vi "Compare to Accel Distances.vi"(5 "dA":dbl, 6 "Sample Period (s)":dbl, 7 "Values":cluster{"accel":dbl, "velocity":dbl}, 8 "Speeds":T1={"maxV (fps)"=20.0, "Accel Limit (fps^2)"=20.0, "Initial V (fps)"=0.0, "Sample Period (s)"=0.02, "Jerk Limit (fps^3)"=0.0, "Front Distances"={"distance (ft)"=0.0, "baseline (ft)"=0.0, "high (ft)"=0.0}, "Back Distances"={"distance (ft)"=0.0, "baseline (ft)"=0.0, "high (ft)"=0.0}}, 10 "Current  Length":dbl, 11 "Total Segment Length":dbl) -> (0 "End Loop":bool, 1 "Ends":cluster{"Accel End":bool, "Decel End":bool}, 2 "Values out":cluster{"accel":dbl, "velocity":dbl}, 3 "Action":enum16{"Const", "Accel", "Decel", "Both"}(ring))   [LabVIEW 2020]
panel:
  out "Accel Action":enum16{"Const", "Accel", "Decel", "Both"}(ring)
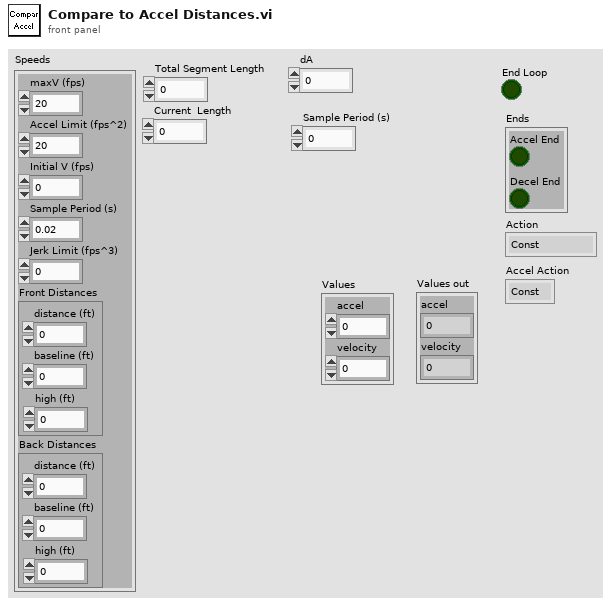
[diagram p1: front panel]
types:
  T1 = cluster{"maxV (fps)":dbl, "Accel Limit (fps^2)":dbl, "Initial V (fps)":dbl, "Sample Period (s)":dbl, "Jerk Limit (fps^3)":dbl, "Front Distances":cluster{"distance (ft)":dbl, "baseline (ft)":dbl, "high (ft)":dbl}, "Back Distances":cluster{"distance (ft)":dbl, "baseline (ft)":dbl, "high (ft)":dbl}}
  T2 = cluster{"distance (ft)":dbl, "baseline (ft)":dbl, "high (ft)":dbl}
  T3 = cluster{"distance (ft)":bool, "baseline (ft)":bool, "high (ft)":bool}
  T4 = cluster{"Accel Limit (fps^2)":dbl, "maxV (fps)":dbl}
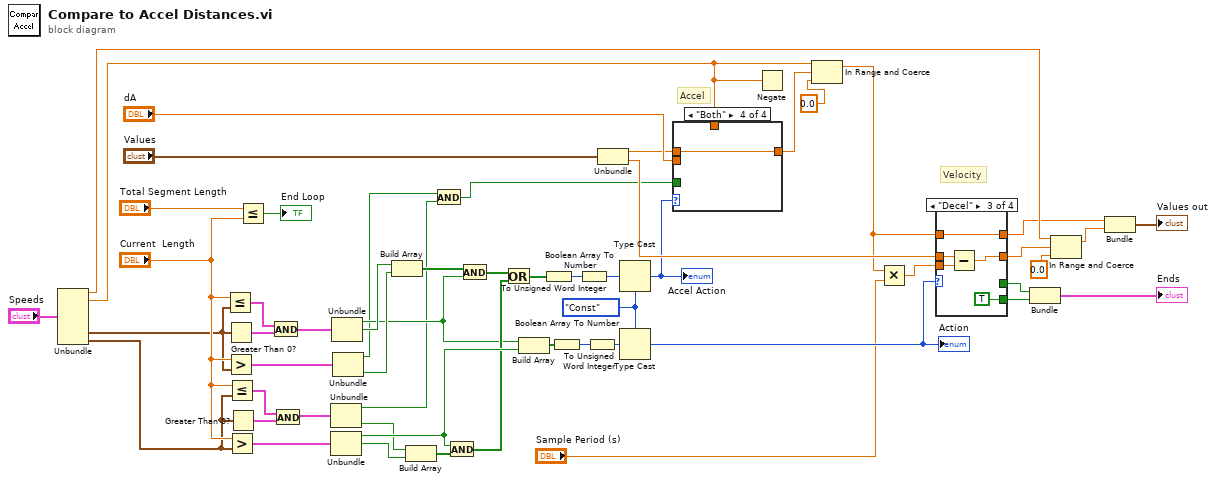
[diagram p0: block diagram]
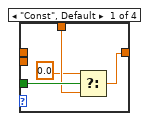
[diagram p2: hidden frame]
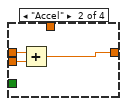
[diagram p3: hidden frame]
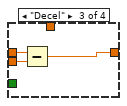
[diagram p4: hidden frame]
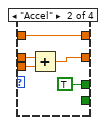
[diagram p6: hidden frame]
diagram:
  w34 = enum16{"Const", "Accel", "Decel", "Both"}."Const" ("Action")
  # "Accel"
  # "Velocity"
  n1 = Unbundle("Speeds") -> ("maxV (fps)"=w9:dbl, "Accel Limit (fps^2)"=w8:dbl, "Front Distances"=w14:T2, "Back Distances"=w13:T2)  [unwired: 3 out]
  n2 = Less Or Equal?(x="Current  Length", y=w14) -> (x <= y?=w52:T3)
  n3 = Greater Than 0?(x=w14) -> (x > 0?=w53:T3)
  n4 = Greater?(x="Current  Length", y=w14) -> (0:w33:T3)
  n5 = Less Or Equal?(x="Current  Length", y=w13) -> (x <= y?=w32:T3)
  n6 = Greater?(x="Current  Length", y=w13) -> (0:w40:T3)
  n7 = Greater Than 0?(x=w13) -> (x > 0?=w31:T3)
  n8 = Less Or Equal?(x="Total Segment Length", y="Current  Length") -> (x <= y?=→"End Loop":bool)
  n9 = And(x=w52, y=w53) -> (x .and. y?=w41:T3)
  n10 = And(x=w32, y=w31) -> (x .and. y?=w28:T3)
  n11 = Unbundle(w28) -> ("distance (ft)"=w2:bool, "high (ft)"=w18:bool)  [unwired: 1 out]
  n12 = Unbundle(w40) -> ("distance (ft)"=w27:bool, "baseline (ft)"=w19:bool)  [unwired: 1 out]
  n13 = Unbundle(w41) -> ("distance (ft)"=w22:bool, "baseline (ft)"=w25:bool)  [unwired: 1 out]
  n14 = Unbundle(w33) -> ("distance (ft)"=w4:bool, "high (ft)"=w29:bool)  [unwired: 1 out]
  n15 = Build Array(w25, w29) -> (w21:bool[])
  n16 = Build Array(w18, w19) -> (w26:bool[])
  n17 = And(x=w4, y=w2) -> (x .and. y?=w3:bool)
  n18 = And(x=w27, y=w26) -> (x .and. y?=w24:bool[])
  n19 = And(x=w21, y=w22) -> (x .and. y?=w20:bool[])
  n20 = Or(x=w20, y=w24) -> (x .or. y?=w23:bool[])
  n21 = Build Array(w22, w27) -> (w42:bool[])
  n22 = Boolean Array To Number(Boolean array=w23) -> (number=w37:u32)
  n23 = Boolean Array To Number(Boolean array=w42) -> (number=w51:u32)
  n24 = To Unsigned Word Integer(number=w37) -> (unsigned 16bit integer=w36:u16)
  n25 = To Unsigned Word Integer(number=w51) -> (unsigned 16bit integer=w39:u16)
  n26 = Unbundle("Values") -> ("accel"=w44:dbl, "velocity"=w43:dbl)
  n27 = Type Cast(type=w34, x=w36) -> (*(type *) &x=w35:enum16{"Const", "Accel", "Decel", "Both"})
  "Accel Action" <- w35
  n28 = Type Cast(type=w34, x=w39) -> (*(type *) &x=w38:enum16{"Const", "Accel", "Decel", "Both"})
  "Action" <- w38
  n29 = case shown="\"Both\"" w35 {
    tunnel: w44 -> [_ w62 w65 w66]
    tunnel: [w56 w60 w63 w66] -> w11
    tunnel: "dA" -> [_ w61 w64 _]
    tunnel: w8 -> [w58 _ _ _]
    tunnel: w3 -> [w59 _ _ _]
    frame "Const", Default {
      n30 = Select(t=0.0, s=w59, f=w58) -> (s? t:f=w56:dbl)
    }
    frame "Accel" {
      n31 = Add(x=w62, y=w61) -> (x+y=w60:dbl)
    }
    frame "Decel" {
      n32 = Subtract(x=w65, y=w64) -> (x-y=w63:dbl)
    }
    frame "Both" {
    }
  }
  n33 = Negate(x=w8) -> ()  [unwired: 1 out]
  n34 = In Range and Coerce(upper limit=w8, x=w11, lower limit=0.0) -> (coerced(x)=w10:dbl)  [unwired: 1 out]
  n35 = Multiply(x=w10, y="Sample Period (s)") -> (x*y=w17:dbl)
  n36 = case shown="\"Decel\"" w38 {
    tunnel: w43 -> [w68 w73 w78 w80]
    tunnel: [w68 w71 w76 w80] -> w7
    tunnel: w17 -> [_ w72 w77 _]
    tunnel: [_ TRUE _ _] -> w48
    tunnel: [_ _ TRUE _] -> w47
    tunnel: [w67 w69 w74 w79] -> w5
    tunnel: w10 -> [w67 w69 w74 w79]
    frame "Const", Default {
    }
    frame "Accel" {
      n37 = Add(x=w73, y=w72) -> (x+y=w71:dbl)
    }
    frame "Decel" {
      n38 = Subtract(x=w78, y=w77) -> (x-y=w76:dbl)
    }
    frame "Both" {
    }
  }
  n39 = Bundle(w48, w47) -> (→"Ends":cluster{bool, bool})  [unwired: 1 in]
  n40 = In Range and Coerce(upper limit=w9, x=w7, lower limit=0.0) -> (coerced(x)=w6:dbl)  [unwired: 1 out]
  n41 = Bundle("Accel Limit (fps^2)"=w5, "maxV (fps)"=w6) -> (→"Values out":T4)  [unwired: 1 in]
